vi "Crossover (Component).vi"(1 "Father":u8[](array[numeric]) format="0x%02x", 2 "Mother":u8[](array[numeric]) format="0x%02x") -> (0 "Child":u8[](array[numeric]) format="0x%02x")   [LabVIEW 2013]
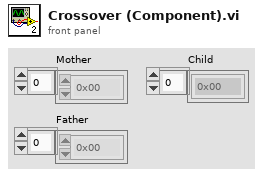
[diagram p1: front panel]
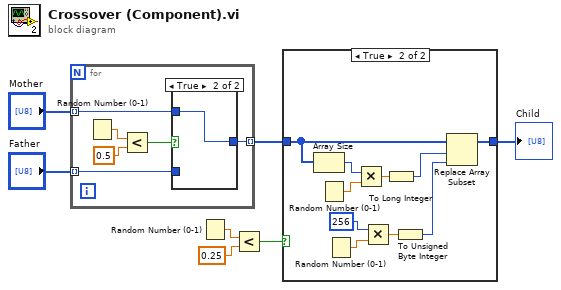
[diagram p0: block diagram]
diagram:
  n1 = for {
    tunnel: "Mother" -> [w9] mode=indexing
    tunnel: "Father" -> [w10] mode=indexing
    tunnel: [w8] -> w5 mode=indexing
    n2 = Random Number (0-1)() -> (number: 0 to 1=w12:dbl)
    n3 = Less?(x=w12, y=0.5) -> (x < y?=w11:bool)
    n4 = case shown="True" w11 {
      tunnel: w10 -> [w14 _]
      tunnel: w9 -> [_ w15]
      tunnel: [w14 w15] -> w8
      frame False {
      }
      frame True {
      }
    }
  }
  n5 = Random Number (0-1)() -> (number: 0 to 1=w4:dbl)
  n6 = Less?(x=w4, y=0.25) -> (x < y?=w2:bool)
  n7 = case shown="True" w2 {
    tunnel: w5 -> [w16 w25]
    tunnel: [w16 w26] -> w1
    frame False {
    }
    frame True {
      n8 = Array Size(array=w25) -> (size(s)=w24:i32)
      n9 = Random Number (0-1)() -> (number: 0 to 1=w23:dbl)
      n10 = Random Number (0-1)() -> (number: 0 to 1=w22:dbl)
      n11 = Multiply(x=w24, y=w23) -> (x*y=w19:dbl)
      n12 = Multiply(x=256, y=w22) -> (x*y=w17:dbl)
      n13 = To Long Integer(number=w19) -> (32bit integer=w18:i32)
      n14 = To Unsigned Byte Integer(number=w17) -> (unsigned 8bit integer=w20:u8)
      n15 = Replace Array Subset(array=w25, new element=w20, index=w18) -> (w26:u8[])
    }
  }
  "Child" <- w1
